vi "写入字节数组.vi"(8 "error in (no error)":errorcluster caption="错误输入（无错误）", 10 "Bytes":u8[](array[numeric]), 11 "串口 输入":refnum<class "串口.lvclass"> caption="DNL_LabVIEW Object in") -> (0 "error out":errorcluster caption="错误输出", 3 "串口 输出":refnum<class "串口.lvclass"> caption="DNL_LabVIEW Object out")   [LabVIEW 2012, in "串口.lvclass"]
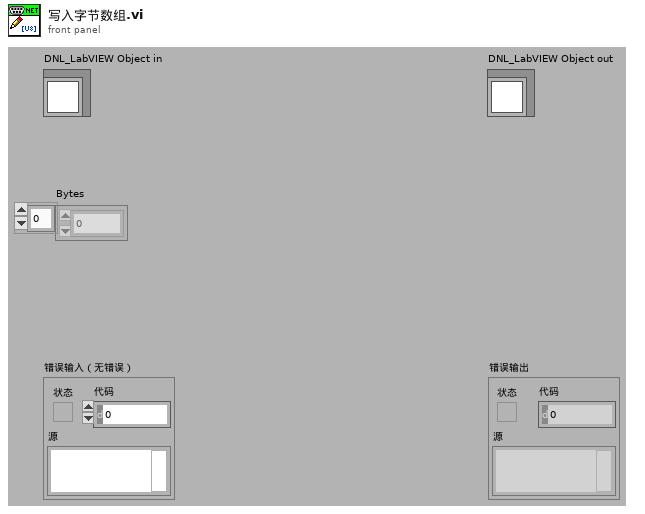
[diagram p1: front panel]
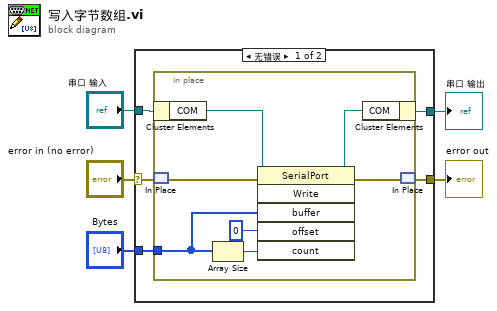
[diagram p0: block diagram]
diagram:
  n1 = case shown="无错误" "error in (no error)" {
    selector: "error in (no error)" -> [w9 w19]
    tunnel: [w8 w19] -> w4
    tunnel: [w6 w18] -> w2
    tunnel: "串口 输入" -> [w10 w18]
    tunnel: "Bytes" -> [w7 _]
    frame No Error {
      n2 = in-place {
        in-place-border: w7 -> [w13]
        n3 = in-place-cluster #1(w10) -> ("COM"=w17:refnum<k24>)
        n4 = in-place-match #2(w9) -> (w16:errorcluster)
        n5 = Array Size(array=w13) -> (size(s)=w12:i32)
        n6 = invoke class="SerialPort" method="Write"(reference=w17, error in=w16, "buffer"=w13, "offset"=0, "count"=w12) -> (reference out=w14:refnum<k24>, error out=w15:errorcluster)  [unwired: 1 in, 4 out]
        n7 = in-place-cluster #1("COM"=w14) -> (w6:refnum<class "串口.lvclass">)
        n8 = in-place-match #2(w15) -> (w8:errorcluster)
      }
    }
    frame Error {
    }
  }
  "error out" <- w4
  "串口 输出" <- w2
